vi "myRIO_BRig_Host_TCP_parseCmd_trial.vi"(10 "input_countCmd":i32, 11 "input_strCmd":string) -> (2 "output_iTrial_num":i32, 3 "output_iTrial_str":string)   [LabVIEW 2014]
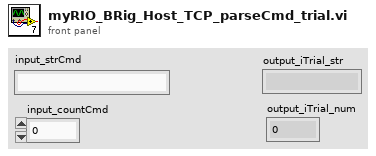
[diagram p1: front panel]
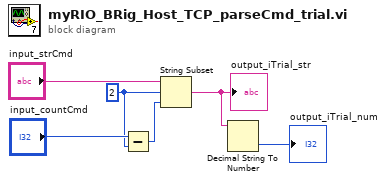
[diagram p0: block diagram]
diagram:
  w4 = 2 ("offset (0)")
  n1 = Subtract(x="input_countCmd", y=w4) -> (x-y=w3:i32)
  n2 = String Subset(string="input_strCmd", offset (0)=w4, length (rest)=w3) -> (substring=w2:string)
  "output_iTrial_str" <- w2
  n3 = Decimal String To Number(string=w2) -> (number=→"output_iTrial_num":i32)  [unwired: 2 in, 1 out]
